vi "oscilloscope.vi"(0 "CH1":bool, 1 "frequency":dbl=10.0 caption="频率" min=0.0 max=1000.0 step=1.0, 2 "频率单位":u16(ring) items=["Hz", "KHz"], 3 "amplitude":dbl=1.0 caption="幅值" min=0.0 max=1000.0 step=1.0 format="%0.2p", 4 "幅值单位":u16(ring) items=["V", "mV"], 5 "phase":dbl caption="相位" format="%.2p", 6 "sampling info":cluster{"Fs":dbl, "#s":dbl}={"Fs"=1000.0, "#s"=1000.0} caption="采样信息" {"Fs" format="%.2p"}) -> ()   [LabVIEW 2020]
uses:
  <vilib>/Analysis/3filter.llb/Filter Passband Type.ctl
  <vilib>/Analysis/3filter.llb/Butterworth Filter (DBL).vi
  <vilib>/measure/mascope.llb/Cycle Average and RMS 1 chan.vi
  <vilib>/measure/matone.llb/Extract Single Tone Information 1 Chan.vi
  <vilib>/measure/NI_MABase.lvlib
  <vilib>/measure/NI_MAPro.lvlib
  <vilib>/Analysis/NI_AALBase.lvlib
panel:
  in  "filter type":T1 caption="滤波器类型"
  in  "order":i32=2 caption="阶数"
  in  "low cutoff freq: fl":dbl=0.12500000000000006 caption="低截止频率:fl" format="%0.4f"
  in  "high cutoff freq: fh":dbl=0.45000000000000007 caption="高截止频率:fh" format="%0.2f"
  in  "选项卡控件":enum32{"示波器", " 滤波器"}(tab)
  out "字符串 2":string
  out "字符串":string
  in  "停止波形":bool
  in  "波形回放":bool
  in  "波形保存":bool
  in  "V-mV":bool
  in  "Hz-KHz":bool
  in  "幅值 v/div":dbl(knob) scale=0.0..4.0
  in  "时间 s/div":dbl(knob) scale=0.0..5.0
  out "频率":dbl format="%.2p"
  out "周期平均":dbl format="%.2p"
  out "周期均方根":dbl format="%.2p"
  out "相位":dbl format="%.2p"
  out "幅度":dbl format="%.2p"
  out "周期平均 2":dbl caption="周期平均" format="%.2p"
  out "周期均方根 2":dbl caption="周期均方根" format="%.2p"
  out "相位 2":dbl caption="相位" format="%.2p"
  out "幅度 2":dbl caption="幅度" format="%.2p"
  out "频率 2":dbl caption="频率" format="%.2p"
  out "波形图":waveform(dbl)[](graph)
  out "波形图 3":dbl[](graph)
  out "波形图 2":dbl[](graph)
  in  "开关":bool
  out "错误输出 2":errorcluster caption="错误输出"
  out "错误输出":errorcluster
  out "波形输出错误":errorcluster
  out "error out 2":errorcluster caption="波形保存错误"
  in  "frequency 2":dbl=10.0 caption="频率" min=0.0 max=1000.0 step=1.0
  in  "频率单位 2":u16(ring) items=["Hz", "KHz"]
  in  "amplitude 2":dbl=1.0 caption="幅值" min=0.0 max=1000.0 step=1.0 format="%0.2p"
  in  "幅值单位  2":u16(ring) items=["V", "mV"]
  in  "phase 2":dbl caption="相位" format="%.2p"
  in  "signal type 2":T2(ring) caption="信号类型"
  in  "CH2":bool
  in  "噪音列表 2":u16(ring) items=["无", "高斯噪音", "均匀白噪音"]
  in  "噪音列表":u16(ring) items=["无", "高斯噪音", "均匀白噪音"]
  out "error out":errorcluster caption="信号发生错误显示"
  in  "signal type":T2(ring) caption="信号类型"
  # "信号发生器"
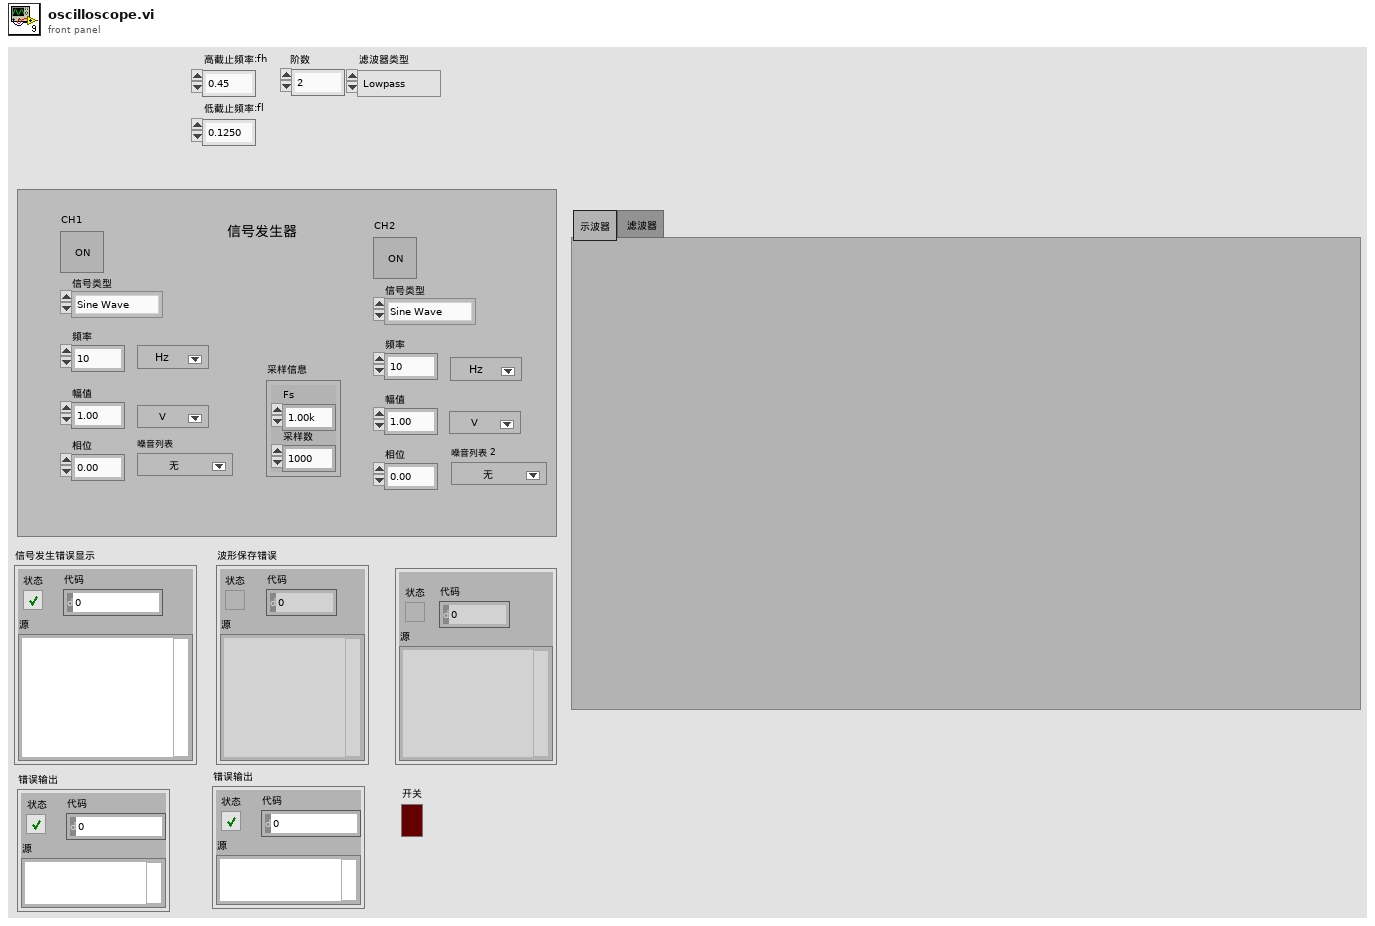
[diagram p1: front panel]
types:
  T1 = typedef "NI_AALBase.lvlib/Filter Passband Type.ctl" = enum32{"Lowpass", "Highpass", "Bandpass", "Bandstop"}
  T2 = enum16{"Sine Wave", "Triangle Wave", "Square Wave", "Sawtooth Wave"}
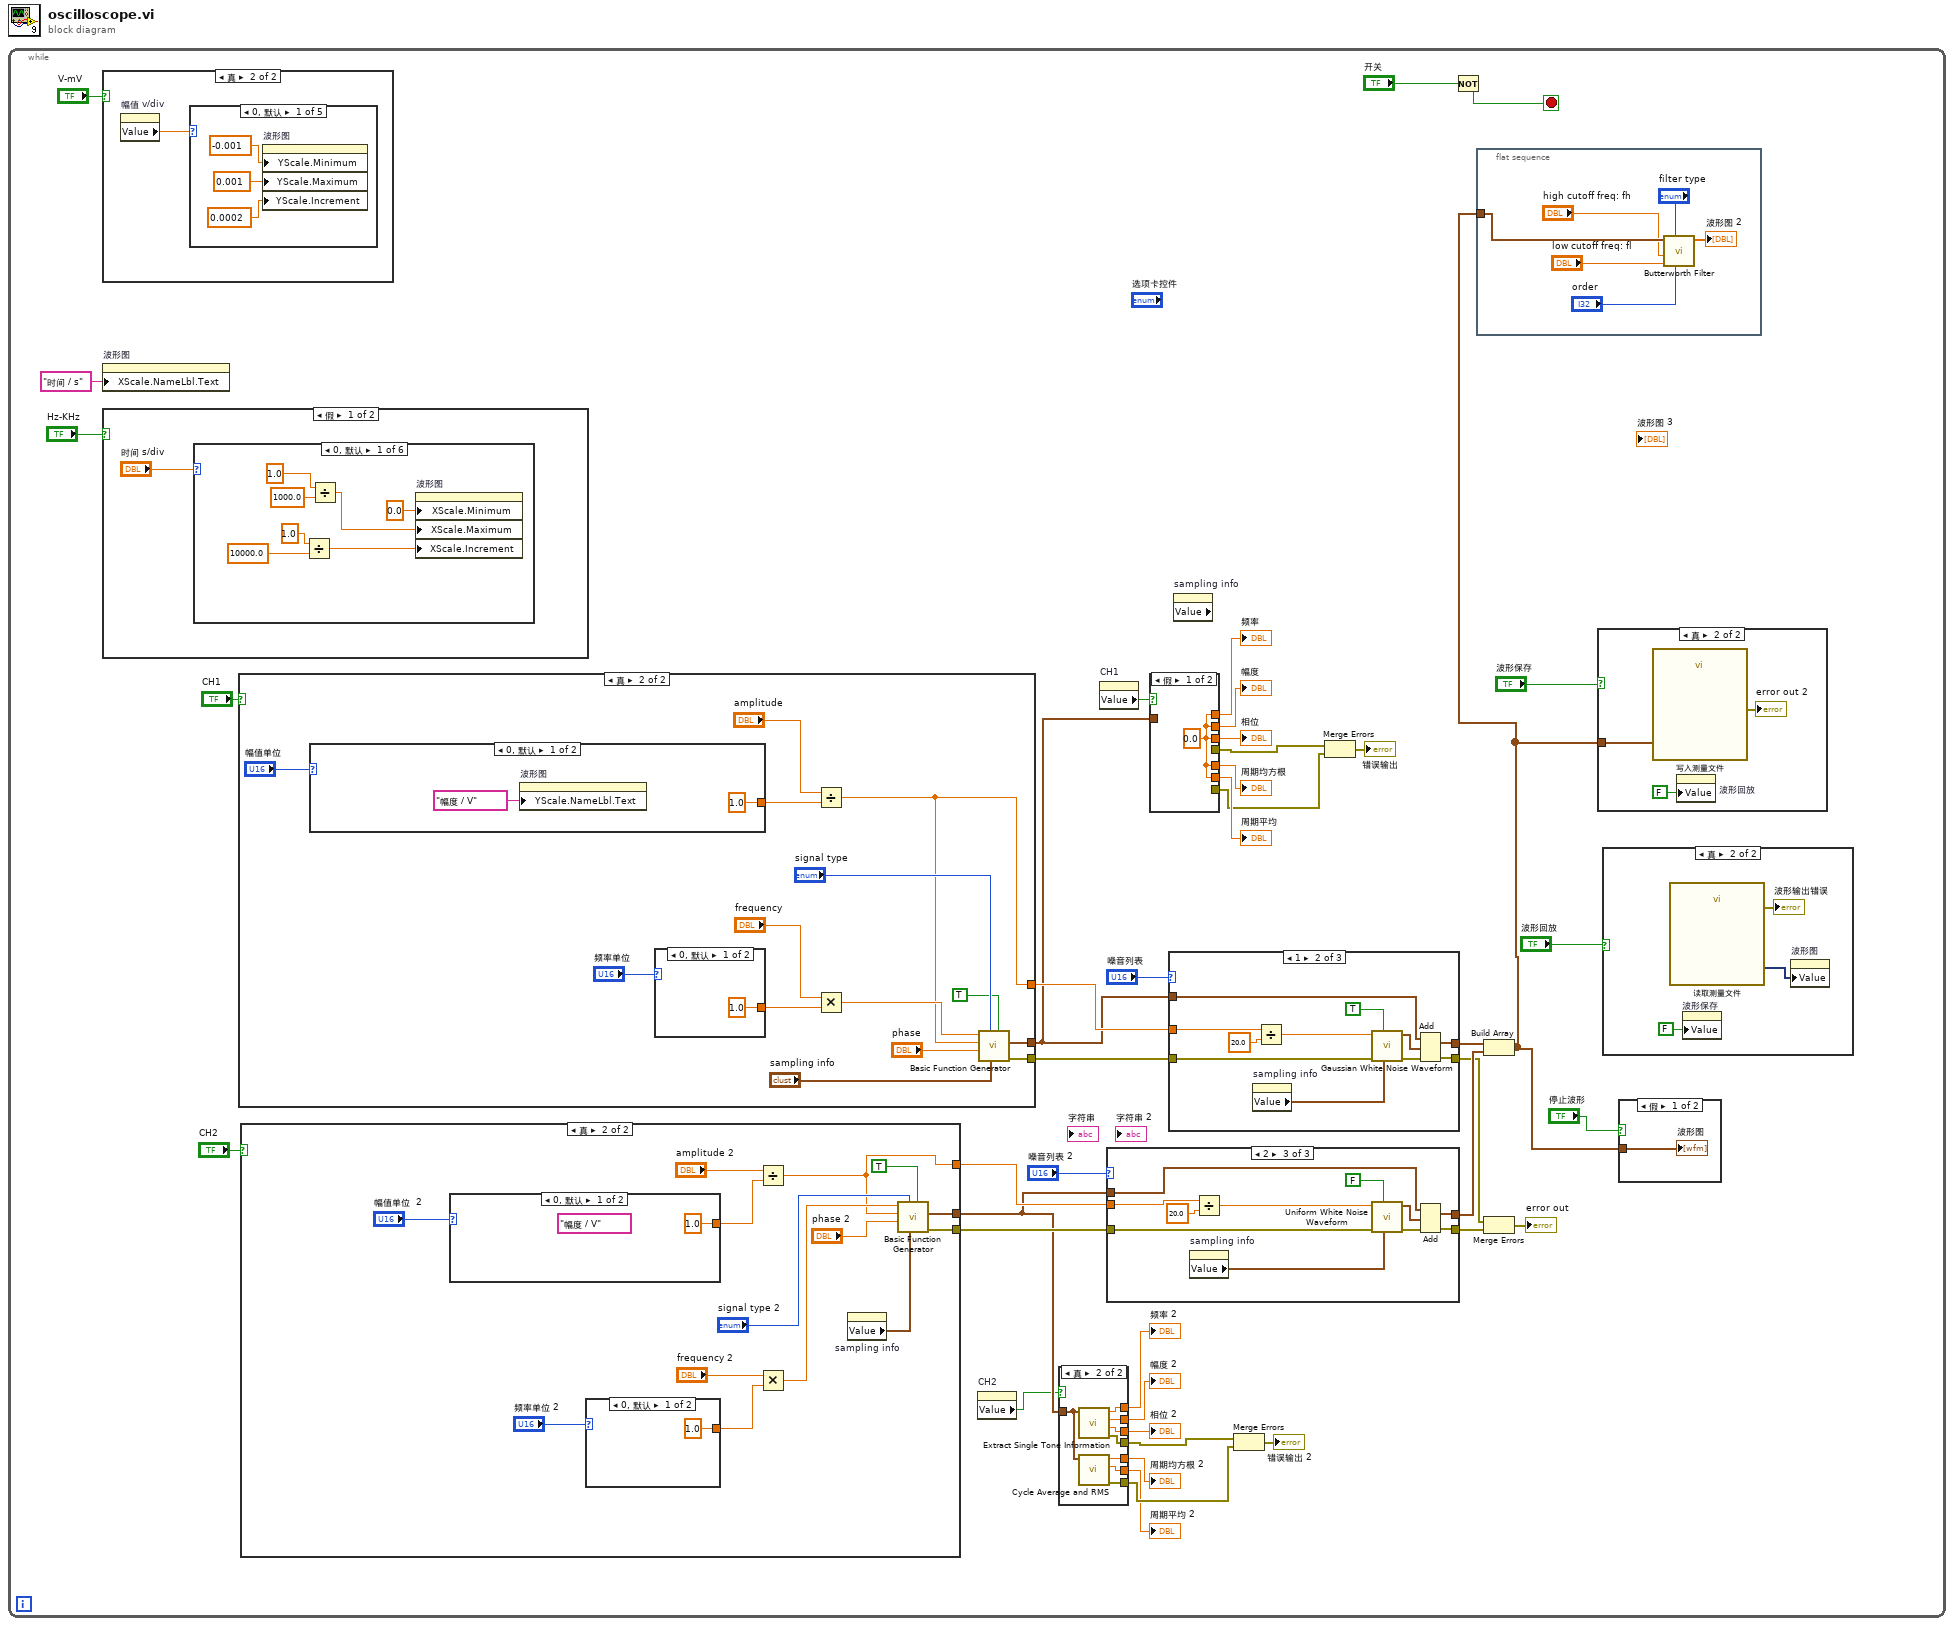
[diagram p0: block diagram]
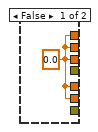
[diagram p2: hidden frame]
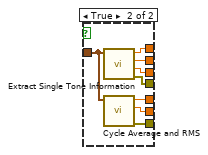
[diagram p3: hidden frame]
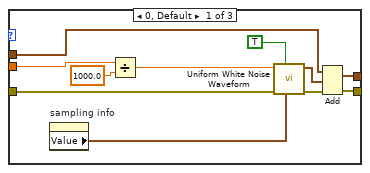
[diagram p7: hidden frame]
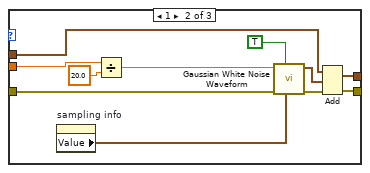
[diagram p8: hidden frame]
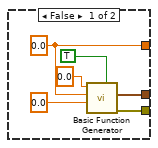
[diagram p9: hidden frame]
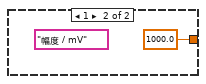
[diagram p10: hidden frame]
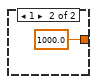
[diagram p11: hidden frame]
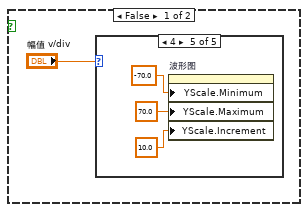
[diagram p12: hidden frame]
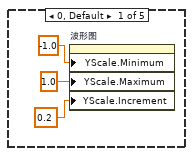
[diagram p13: hidden frame]
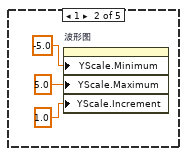
[diagram p14: hidden frame]
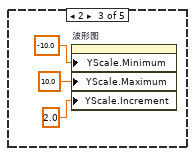
[diagram p15: hidden frame]
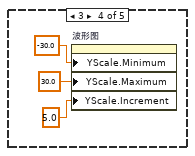
[diagram p16: hidden frame]
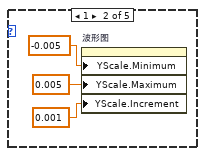
[diagram p17: hidden frame]
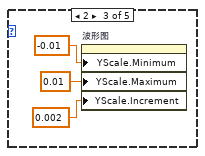
[diagram p18: hidden frame]
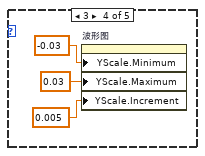
[diagram p19: hidden frame]
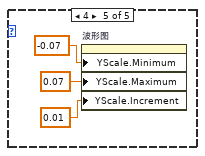
[diagram p20: hidden frame]
diagram:
  n1 = while {
    stop <- w40 stop-if-true
    n2 = case shown="真" "V-mV" {
      frame False {
        n3 = case shown="4" "幅值 v/div" {
          frame 0, Default {
            n4 = property on="波形图" class="WFGraph (严格)"("YScale.Minimum"=-1.0 ("Y标尺.范围:最小值"), "YScale.Maximum"=1.0 ("Y标尺.范围:最大值"), "YScale.Increment"=0.2 ("Y标尺.范围:增量")) -> ()  [unwired: 2 in, 2 out]
          }
          frame 1 {
            n5 = property on="波形图" class="WFGraph (严格)"("YScale.Minimum"=-5.0 ("Y标尺.范围:最小值"), "YScale.Maximum"=5.0 ("Y标尺.范围:最大值"), "YScale.Increment"=1.0 ("Y标尺.范围:增量")) -> ()  [unwired: 2 in, 2 out]
          }
          frame 2 {
            n6 = property on="波形图" class="WFGraph (严格)"("YScale.Minimum"=-10.0 ("Y标尺.范围:最小值"), "YScale.Maximum"=10.0 ("Y标尺.范围:最大值"), "YScale.Increment"=2.0 ("Y标尺.范围:增量")) -> ()  [unwired: 2 in, 2 out]
          }
          frame 3 {
            n7 = property on="波形图" class="WFGraph (严格)"("YScale.Minimum"=-30.0 ("Y标尺.范围:最小值"), "YScale.Maximum"=30.0 ("Y标尺.范围:最大值"), "YScale.Increment"=5.0 ("Y标尺.范围:增量")) -> ()  [unwired: 2 in, 2 out]
          }
          frame 4 {
            n8 = property on="波形图" class="WFGraph (严格)"("YScale.Minimum"=-70.0 ("Y标尺.范围:最小值"), "YScale.Maximum"=70.0 ("Y标尺.范围:最大值"), "YScale.Increment"=10.0 ("Y标尺.范围:增量")) -> ()  [unwired: 2 in, 2 out]
          }
        }
      }
      frame True {
        n9 = property on="幅值 v/div" class="Knob (严格)"() -> ("Value"=w147:dbl)  [unwired: 2 in, 2 out]
        n10 = case shown="0, 默认" w147 {
          frame 0, Default {
            n11 = property on="波形图" class="WFGraph (严格)"("YScale.Minimum"=-0.001 ("Y标尺.范围:最小值"), "YScale.Maximum"=0.001 ("Y标尺.范围:最大值"), "YScale.Increment"=0.0002 ("Y标尺.范围:增量")) -> ()  [unwired: 2 in, 2 out]
          }
          frame 1 {
            n12 = property on="波形图" class="WFGraph (严格)"("YScale.Minimum"=-0.005 ("Y标尺.范围:最小值"), "YScale.Maximum"=0.005 ("Y标尺.范围:最大值"), "YScale.Increment"=0.001 ("Y标尺.范围:增量")) -> ()  [unwired: 2 in, 2 out]
          }
          frame 2 {
            n13 = property on="波形图" class="WFGraph (严格)"("YScale.Minimum"=-0.01 ("Y标尺.范围:最小值"), "YScale.Maximum"=0.01 ("Y标尺.范围:最大值"), "YScale.Increment"=0.002 ("Y标尺.范围:增量")) -> ()  [unwired: 2 in, 2 out]
          }
          frame 3 {
            n14 = property on="波形图" class="WFGraph (严格)"("YScale.Minimum"=-0.03 ("Y标尺.范围:最小值"), "YScale.Maximum"=0.03 ("Y标尺.范围:最大值"), "YScale.Increment"=0.005 ("Y标尺.范围:增量")) -> ()  [unwired: 2 in, 2 out]
          }
          frame 4 {
            n15 = property on="波形图" class="WFGraph (严格)"("YScale.Minimum"=-0.07 ("Y标尺.范围:最小值"), "YScale.Maximum"=0.07 ("Y标尺.范围:最大值"), "YScale.Increment"=0.01 ("Y标尺.范围:增量")) -> ()  [unwired: 2 in, 2 out]
          }
        }
      }
    }
    n16 = property on="波形图" class="WFGraph (严格)"("XScale.NameLbl.Text"="时间 / s" ("X标尺.名称标签.文本")) -> ()  [unwired: 2 in, 2 out]
    n17 = case shown="假" "Hz-KHz" {
      frame False {
        n18 = case shown="0, 默认" "时间 s/div" {
          frame 0, Default {
            n19 = Divide(x=1.0, y=10000.0) -> (x/y=w164:dbl)
            n20 = Divide(x=1.0, y=1000.0) -> (x/y=w167:dbl)
            n21 = property on="波形图" class="WFGraph (严格)"("XScale.Minimum"=0.0 ("X标尺.范围:最小值"), "XScale.Maximum"=w167, "XScale.Increment"=w164) -> ()  [unwired: 2 in, 2 out]
          }
          frame 1 {
            n22 = Divide(x=1.0, y=1000.0) -> (x/y=w171:dbl)
            n23 = Divide(x=1.0, y=100.0) -> (x/y=w174:dbl)
            n24 = property on="波形图" class="WFGraph (严格)"("XScale.Minimum"=0.0 ("X标尺.范围:最小值"), "XScale.Maximum"=w174, "XScale.Increment"=w171) -> ()  [unwired: 2 in, 2 out]
          }
          frame 2 {
            n25 = Divide(x=5.0, y=1000.0) -> (x/y=w178:dbl)
            n26 = Divide(x=5.0, y=100.0) -> (x/y=w181:dbl)
            n27 = property on="波形图" class="WFGraph (严格)"("XScale.Minimum"=0.0 ("X标尺.范围:最小值"), "XScale.Maximum"=w181, "XScale.Increment"=w178) -> ()  [unwired: 2 in, 2 out]
          }
          frame 3 {
            n28 = Divide(x=1.0, y=10.0) -> (x/y=w188:dbl)
            n29 = Divide(x=1.0, y=100.0) -> (x/y=w185:dbl)
            n30 = property on="波形图" class="WFGraph (严格)"("XScale.Minimum"=0.0 ("X标尺.范围:最小值"), "XScale.Maximum"=w188, "XScale.Increment"=w185) -> ()  [unwired: 2 in, 2 out]
          }
          frame 4 {
            n31 = Divide(x=15.0, y=1000.0) -> (x/y=w192:dbl)
            n32 = Divide(x=15.0, y=100.0) -> (x/y=w195:dbl)
            n33 = property on="波形图" class="WFGraph (严格)"("XScale.Minimum"=0.0 ("X标尺.范围:最小值"), "XScale.Maximum"=w195, "XScale.Increment"=w192) -> ()  [unwired: 2 in, 2 out]
          }
          frame 5 {
            n34 = Divide(x=2.0, y=10.0) -> (x/y=w205:dbl)
            n35 = Divide(x=2.0, y=100.0) -> (x/y=w204:dbl)
            n36 = property on="波形图" class="WFGraph (严格)"("XScale.Minimum"=0.0 ("X标尺.范围:最小值"), "XScale.Maximum"=w205, "XScale.Increment"=w204) -> ()  [unwired: 2 in, 2 out]
          }
        }
      }
      frame True {
        n37 = property on="时间 s/div" class="Knob (严格)"() -> ("Value"=w206:dbl)  [unwired: 2 in, 2 out]
        n38 = case shown="4" w206 {
          frame 0, Default {
            n39 = Divide(x=1.0, y=1000000.0) -> (x/y=w210:dbl)
            n40 = Divide(x=1.0, y=10000000.0) -> (x/y=w207:dbl)
            n41 = property on="波形图" class="WFGraph (严格)"("XScale.Minimum"=0.0 ("X标尺.范围:最小值"), "XScale.Maximum"=w210, "XScale.Increment"=w207) -> ()  [unwired: 2 in, 2 out]
          }
          frame 1 {
            n42 = Divide(x=1.0, y=100000.0) -> (x/y=w217:dbl)
            n43 = Divide(x=1.0, y=1000000.0) -> (x/y=w214:dbl)
            n44 = property on="波形图" class="WFGraph (严格)"("XScale.Minimum"=0.0 ("X标尺.范围:最小值"), "XScale.Maximum"=w217, "XScale.Increment"=w214) -> ()  [unwired: 2 in, 2 out]
          }
          frame 2 {
            n45 = Divide(x=5.0, y=100000.0) -> (x/y=w224:dbl)
            n46 = Divide(x=5.0, y=1000000.0) -> (x/y=w221:dbl)
            n47 = property on="波形图" class="WFGraph (严格)"("XScale.Minimum"=0.0 ("X标尺.范围:最小值"), "XScale.Maximum"=w224, "XScale.Increment"=w221) -> ()  [unwired: 2 in, 2 out]
          }
          frame 3 {
            n48 = Divide(x=1.0, y=10000.0) -> (x/y=w231:dbl)
            n49 = Divide(x=1.0, y=100000.0) -> (x/y=w228:dbl)
            n50 = property on="波形图" class="WFGraph (严格)"("XScale.Minimum"=0.0 ("X标尺.范围:最小值"), "XScale.Maximum"=w231, "XScale.Increment"=w228) -> ()  [unwired: 2 in, 2 out]
          }
          frame 4 {
            n51 = Divide(x=15.0, y=100000.0) -> (x/y=w238:dbl)
            n52 = Divide(x=15.0, y=1000000.0) -> (x/y=w235:dbl)
            n53 = property on="波形图" class="WFGraph (严格)"("XScale.Minimum"=0.0 ("X标尺.范围:最小值"), "XScale.Maximum"=w238, "XScale.Increment"=w235) -> ()  [unwired: 2 in, 2 out]
          }
          frame 5 {
            n54 = Divide(x=2.0, y=10000.0) -> (x/y=w248:dbl)
            n55 = Divide(x=2.0, y=100000.0) -> (x/y=w247:dbl)
            n56 = property on="波形图" class="WFGraph (严格)"("XScale.Minimum"=0.0 ("X标尺.范围:最小值"), "XScale.Maximum"=w248, "XScale.Increment"=w247) -> ()  [unwired: 2 in, 2 out]
          }
        }
      }
    }
    n57 = case shown="真" "CH1" {
      tunnel: [w285 w291] -> w21
      tunnel: [w284 w290] -> w38
      tunnel: [w283 w289] -> w37
      frame False {
        w283 = 0.0 ("amplitude")
        n58 = property on="sampling info" class="Clust (严格)"() -> ("Value"=w282:cluster{"Fs":dbl, "#s":dbl})  [unwired: 2 in, 2 out]
        n59 = call <vilib>:"Basic Function Generator.vi"("reset signal"=TRUE, "sampling info"=w282, "phase"=0.0, "amplitude"=w283, "frequency"=0.0) -> ("error out"=w284:errorcluster, "signal out"=w285:waveform(dbl))  [unwired: 4 in, 1 out]
      }
      frame True {
        n60 = case shown="0, 默认" "幅值单位" {
          tunnel: [1.0 1000.0] -> w295
          frame 0, Default {
            n61 = property on="波形图" class="WFGraph (严格)"("YScale.NameLbl.Text"="幅度 / V") -> ()  [unwired: 2 in, 2 out]
          }
          frame 1 {
            n62 = property on="波形图" class="WFGraph (严格)"("YScale.NameLbl.Text"="幅度 / mV") -> ()  [unwired: 2 in, 2 out]
          }
        }
        n63 = case shown="0, 默认" "频率单位" {
          tunnel: [1.0 1000.0] -> w300
          frame 0, Default {
          }
          frame 1 {
          }
        }
        n64 = Divide(x="amplitude", y=w295) -> (x/y=w289:dbl)
        n65 = Multiply(x="frequency", y=w300) -> (x*y=w299:dbl)
        n66 = call <vilib>:"Basic Function Generator.vi"("reset signal"=TRUE, "sampling info"="sampling info", "signal type"="signal type", "phase"="phase", "amplitude"=w289, "frequency"=w299) -> ("error out"=w290:errorcluster, "signal out"=w291:waveform(dbl))  [unwired: 3 in, 1 out]
      }
    }
    n67 = case shown="真" "CH2" {
      tunnel: [w109 w116] -> w3
      tunnel: [w108 w115] -> w32
      tunnel: [w107 w114] -> w33
      frame False {
        w107 = 0.0 ("amplitude")
        n68 = call <vilib>:"Basic Function Generator.vi"("reset signal"=TRUE, "phase"=0.0, "amplitude"=w107, "frequency"=0.0) -> ("error out"=w108:errorcluster, "signal out"=w109:waveform(dbl))  [unwired: 5 in, 1 out]
      }
      frame True {
        n69 = case shown="0, 默认" "幅值单位  2" {
          tunnel: [1.0 1000.0] -> w120
          frame 0, Default {
            (unwired) "幅度 / V"
          }
          frame 1 {
            (unwired) "幅度 / mV"
          }
        }
        n70 = case shown="0, 默认" "频率单位 2" {
          tunnel: [1.0 1000.0] -> w124
          frame 0, Default {
          }
          frame 1 {
          }
        }
        n71 = Divide(x="amplitude 2", y=w120) -> (x/y=w114:dbl)
        n72 = Multiply(x="frequency 2", y=w124) -> (x*y=w123:dbl)
        n73 = property on="sampling info" class="Clust (严格)"() -> ("Value"=w113:cluster{"Fs":dbl, "#s":dbl})  [unwired: 2 in, 2 out]
        n74 = call <vilib>:"Basic Function Generator.vi"("reset signal"=TRUE, "sampling info"=w113, "signal type"="signal type 2", "phase"="phase 2", "amplitude"=w114, "frequency"=w123) -> ("error out"=w115:errorcluster, "signal out"=w116:waveform(dbl))  [unwired: 3 in, 1 out]
      }
    }
    n75 = property on="CH2" class="Bool (严格)"() -> ("Value"=w2:bool)  [unwired: 2 in, 2 out]
    n76 = case shown="真" w2 {
      tunnel: w3 -> [_ w57]
      tunnel: [w49 w56] -> w4
      tunnel: [w49 w55] -> w5
      tunnel: [w49 w54] -> w6
      tunnel: [w49 w53] -> w7
      tunnel: [w49 w52] -> w8
      tunnel: [_ w51] -> w9
      tunnel: [_ w50] -> w10
      frame False {
        w49 = 0.0
      }
      frame True {
        n77 = call-poly <vilib>:"Extract Single Tone Information.vi"("time signal in"=w57) -> ("error out"=w51:errorcluster, "detected phase (deg)"=w54:dbl, "detected amplitude"=w55:dbl, "detected frequency"=w56:dbl)  [unwired: 5 in, 2 out]
        n78 = call-poly <vilib>:"Cycle Average and RMS.vi"("signal in"=w57) -> ("error out"=w50:errorcluster, "cycle RMS"=w52:dbl, "cycle average"=w53:dbl)  [unwired: 7 in, 1 out]
      }
    }
    "频率 2" <- w4
    "幅度 2" <- w5
    "相位 2" <- w6
    "周期均方根 2" <- w7
    "周期平均 2" <- w8
    n79 = property on="CH1" class="Bool (严格)"() -> ("Value"=w20:bool)  [unwired: 2 in, 2 out]
    n80 = case shown="2" "噪音列表 2" {
      tunnel: w3 -> [w79 w90 w102]
      tunnel: w32 -> [w76 w88 w99]
      tunnel: w33 -> [w83 w94 w105]
      tunnel: [w78 w89 w101] -> w29
      tunnel: [w75 w86 w97] -> w27
      frame 0, Default {
        n81 = property on="sampling info" class="Clust (严格)"() -> ("Value"=w74:cluster{"Fs":dbl, "#s":dbl})  [unwired: 2 in, 2 out]
        n82 = Divide(x=w83, y=1000.0) -> (x/y=w81:dbl)
        n83 = call <vilib>:"Uniform White Noise Waveform.vi"("sampling info"=w74, "reset signal"=TRUE, "error in (no error)"=w76, "amplitude"=w81) -> ("error out"=w77:errorcluster, "signal out"=w80:waveform(dbl))  [unwired: 6 in]
        n84 = Add(1:w80, 2:w79, 4:w77) -> (0:w78:waveform(dbl), 3:w75:errorcluster)
      }
      frame 1 {
        n85 = property on="sampling info" class="Clust (严格)"() -> ("Value"=w85:cluster{"Fs":dbl, "#s":dbl})  [unwired: 2 in, 2 out]
        n86 = Divide(x=w94, y=20.0) -> (x/y=w92:dbl)
        n87 = call <vilib>:"Gaussian White Noise Waveform.vi"("sampling info"=w85, "reset signal"=TRUE, "error in (no error)"=w88, "standard deviation"=w92) -> ("error out"=w87:errorcluster, "signal out"=w91:waveform(dbl))  [unwired: 6 in]
        n88 = Add(1:w91, 2:w90, 4:w87) -> (0:w89:waveform(dbl), 3:w86:errorcluster)
      }
      frame 2 {
        n89 = property on="sampling info" class="Clust (严格)"() -> ("Value"=w96:cluster{"Fs":dbl, "#s":dbl})  [unwired: 2 in, 2 out]
        n90 = Divide(x=w105, y=20.0) -> (x/y=w103:dbl)
        n91 = call <vilib>:"Uniform White Noise Waveform.vi"("sampling info"=w96, "reset signal"=FALSE, "error in (no error)"=w99, "amplitude"=w103) -> ("error out"=w98:errorcluster, "signal out"=w100:waveform(dbl))  [unwired: 6 in]
        n92 = Add(1:w100, 2:w102, 4:w98) -> (0:w101:waveform(dbl), 3:w97:errorcluster)
      }
    }
    n93 = case shown="假" w20 {
      tunnel: w21 -> [_ w66]
      tunnel: [w58 w65] -> w19
      tunnel: [w58 w64] -> w18
      tunnel: [w58 w63] -> w17
      tunnel: [w58 w62] -> w16
      tunnel: [w58 w61] -> w15
      tunnel: [_ w60] -> w14
      tunnel: [_ w59] -> w13
      frame False {
        w58 = 0.0
      }
      frame True {
        n94 = call-poly <vilib>:"Extract Single Tone Information.vi"("time signal in"=w66) -> ("error out"=w60:errorcluster, "detected phase (deg)"=w63:dbl, "detected amplitude"=w64:dbl, "detected frequency"=w65:dbl)  [unwired: 5 in, 2 out]
        n95 = call-poly <vilib>:"Cycle Average and RMS.vi"("signal in"=w66) -> ("error out"=w59:errorcluster, "cycle RMS"=w61:dbl, "cycle average"=w62:dbl)  [unwired: 7 in, 1 out]
      }
    }
    "频率" <- w19
    "幅度" <- w18
    "相位" <- w17
    "周期均方根" <- w16
    "周期平均" <- w15
    n96 = case shown="1" "噪音列表" {
      tunnel: w21 -> [w254 w265 w277]
      tunnel: w38 -> [w251 w263 w274]
      tunnel: w37 -> [w258 w269 w280]
      tunnel: [w253 w264 w276] -> w28
      tunnel: [w250 w261 w272] -> w26
      frame 0, Default {
        n97 = property on="sampling info" class="Clust (严格)"() -> ("Value"=w249:cluster{"Fs":dbl, "#s":dbl})  [unwired: 2 in, 2 out]
        n98 = Divide(x=w258, y=1000.0) -> (x/y=w256:dbl)
        n99 = call <vilib>:"Uniform White Noise Waveform.vi"("sampling info"=w249, "reset signal"=TRUE, "error in (no error)"=w251, "amplitude"=w256) -> ("error out"=w252:errorcluster, "signal out"=w255:waveform(dbl))  [unwired: 6 in]
        n100 = Add(1:w255, 2:w254, 4:w252) -> (0:w253:waveform(dbl), 3:w250:errorcluster)
      }
      frame 1 {
        n101 = property on="sampling info" class="Clust (严格)"() -> ("Value"=w260:cluster{"Fs":dbl, "#s":dbl})  [unwired: 2 in, 2 out]
        n102 = Divide(x=w269, y=20.0) -> (x/y=w267:dbl)
        n103 = call <vilib>:"Gaussian White Noise Waveform.vi"("sampling info"=w260, "reset signal"=TRUE, "error in (no error)"=w263, "standard deviation"=w267) -> ("error out"=w262:errorcluster, "signal out"=w266:waveform(dbl))  [unwired: 6 in]
        n104 = Add(1:w266, 2:w265, 4:w262) -> (0:w264:waveform(dbl), 3:w261:errorcluster)
      }
      frame 2 {
        n105 = property on="sampling info" class="Clust (严格)"() -> ("Value"=w271:cluster{"Fs":dbl, "#s":dbl})  [unwired: 2 in, 2 out]
        n106 = Divide(x=w280, y=20.0) -> (x/y=w278:dbl)
        n107 = call <vilib>:"Uniform White Noise Waveform.vi"("sampling info"=w271, "reset signal"=FALSE, "error in (no error)"=w274, "amplitude"=w278) -> ("error out"=w273:errorcluster, "signal out"=w275:waveform(dbl))  [unwired: 6 in]
        n108 = Add(1:w275, 2:w277, 4:w273) -> (0:w276:waveform(dbl), 3:w272:errorcluster)
      }
    }
    n109 = property on="sampling info" class="Clust (严格)" props=["Value"]() -> ()  [unwired: 2 in, 3 out]
    n110 = Merge Errors(w9, w10) -> (→"错误输出 2":errorcluster)
    n111 = Merge Errors(w14, w13) -> (→"错误输出":errorcluster)
    n112 = Not(x="开关") -> (.not. x?=w40:bool)
    n113 = flat-sequence {
      tunnel: w1 -> [w48]
      frame #0 {
        n114 = call-poly <vilib>:"Butterworth Filter.vi"("order"="order", "filter type"="filter type", "low cutoff freq: fl"="low cutoff freq: fl", "high cutoff freq: fh"="high cutoff freq: fh", "X"=w48) -> ("Filtered X"=→"波形图 2":dbl[])  [unwired: 3 in, 1 out]
      }
    }
    n115 = Build Array(w28, w29) -> (w1:waveform(dbl)[])
    n116 = Merge Errors(w26, w27) -> (→"error out":errorcluster)
    n117 = case shown="真" "波形保存" {
      tunnel: w1 -> [_ w73]
      frame False {
      }
      frame True {
        n118 = call "写入测量文件"("Signals"=w73) -> ("error out"=→"error out 2":errorcluster)  [unwired: 16 in, 2 out]
        n119 = property on="波形回放" class="Bool (严格)"("Value"=FALSE ("波形回放")) -> ()  [unwired: 2 in, 2 out]
      }
    }
    n120 = case shown="真" "波形回放" {
      frame False {
      }
      frame True {
        n121 = call "读取测量文件"() -> ("error out"=→"波形输出错误":errorcluster, "Signals"=w69:dynamicdata)  [unwired: 6 in, 4 out]
        n122 = property on="波形保存" class="Bool (严格)"("Value"=FALSE ("波形保存")) -> ()  [unwired: 2 in, 2 out]
        n123 = property on="波形图" class="WFGraph (严格)"("Value"=w69) -> ()  [unwired: 2 in, 2 out]
      }
    }
    n124 = case shown="假" "停止波形" {
      tunnel: w1 -> [w67 _]
      frame False {
        "波形图" <- w67
      }
      frame True {
      }
    }
  }
